vi "Build Standard Bus Register Look Up Table--VI.vi"(8 "error in":errorcluster, 11 "Spreadsheet Path":path=path "C:/Repos/thermal-chamber-module/Libraries/Thermal Chamber/Documentation/Standard Bus Registers.csv") -> (0 "error out":errorcluster)   [LabVIEW 2024, in "Watlow F4T.lvclass"]
uses:
  Watlow F4T.lvclass
  <vilib>/Utility/file.llb/Read Delimited Spreadsheet (string).vi
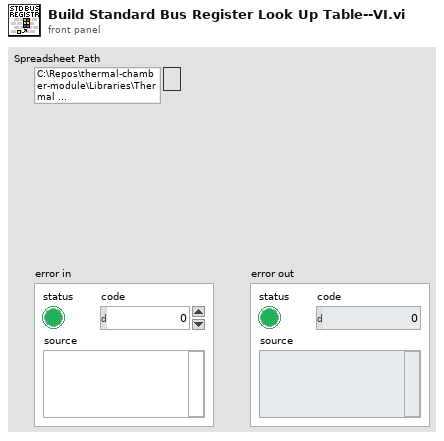
[diagram p1: front panel]
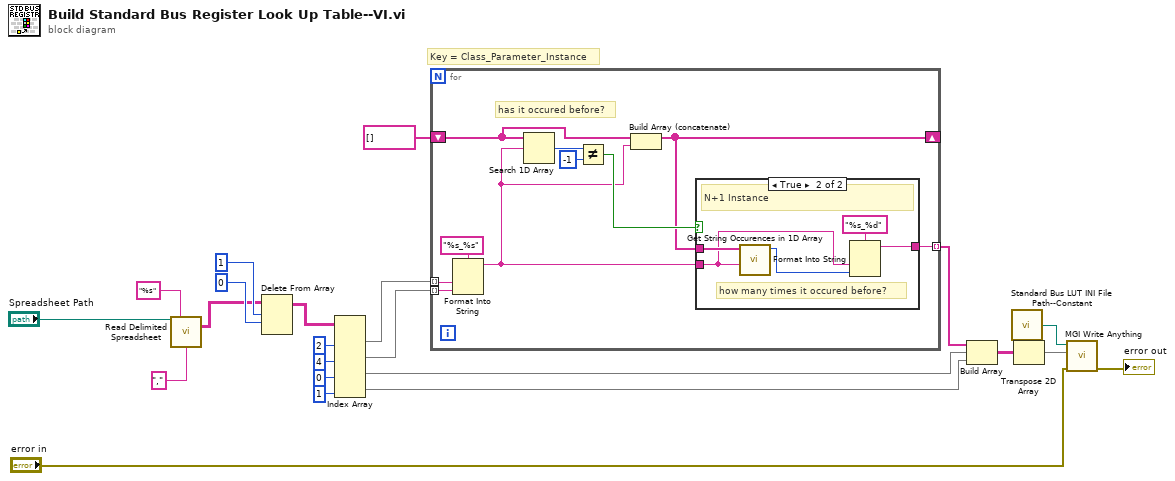
[diagram p0: block diagram]
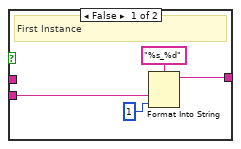
[diagram p2: hidden frame]
diagram:
  # "Key = Class_Parameter_Instance"
  n1 = call-poly <vilib>:"Read Delimited Spreadsheet.vi"("file path (dialog if empty)"="Spreadsheet Path", "format (%s)"="%s", "delimiter (\\t)"="," ("delimiter (\\t)")) -> ("all rows"=w6:string[][])  [unwired: 7 in, 5 out]
  n2 = Delete From Array(array=w6, length=1, index (row)=0) -> (array with subset deleted=w9:string[][])  [unwired: 1 in, 1 out]
  n3 = Index Array(array=w9, index (col) #1=2 ("disabled index (col)"), index (col) #2=4 ("index (col)"), index (col) #3=0 ("index (col)"), index (col) #4=1 ("index (col)")) -> (element #1=w16:string[], element #2=w17:string[], element #3=w14:string[], element #4=w15:string[])  [unwired: 4 in]
  n4 = for {
    tunnel: w16 -> [w30] mode=indexing
    tunnel: w17 -> [w31] mode=indexing
    shift-right: [w23] -> _
    shift-left: string[] [] -> [w26]
    tunnel: [w25] -> w19 mode=indexing
    # "has it occured before?"
    n5 = Format Into String(format string="%s_%s", w30, w31) -> (resulting string=w24:string)  [unwired: 2 in, 1 out]
    n6 = Search 1D Array(1D array=w26, element=w24) -> (index of element=w29:i32)  [unwired: 1 in]
    n7 = Not Equal?(x=w29, y=-1) -> (x != y?=w27:bool)
    n8 = Build Array (concatenate)(w26, w24) -> (w23:string[])
    n9 = case shown="True" w27 {
      tunnel: w24 -> [w35 w38]
      tunnel: [w33 w40] -> w25
      tunnel: w23 -> [_ w39]
      frame False {
        # "First Instance"
        n10 = Format Into String(format string="%s_%d", w35, 1 ("input 2")) -> (resulting string=w33:string)  [unwired: 2 in, 1 out]
      }
      frame True {
        # "how many times it occured before?"
        # "N+1 Instance"
        n11 = call "Get String Occurences in 1D Array.vi"("Search String"=w38, "Array of Strings"=w39) -> ("# of Occurences"=w37:i32)  [unwired: 9 in]
        n12 = Format Into String(format string="%s_%d", w38, w37) -> (resulting string=w40:string)  [unwired: 2 in, 1 out]
      }
    }
  }
  n13 = Build Array(w19, w14, w15) -> (w20:string[][])
  n14 = call "Standard Bus LUT INI File Path--Constant.vi"() -> ("Standard Bus Register LUT Path"=w1:path)  [unwired: 1 in]
  n15 = Transpose 2D Array(2D array=w20) -> (transposed array=w21:string[][])
  n16 = call <userlib>:"MGI Write Anything.vi"("Error In"="error in", "Anything"=w21, "Path (dialog)"=w1) -> ("Error Out"=→"error out":errorcluster)  [unwired: 6 in, 2 out]
